vi "init stack.vi"() -> ()   [LabVIEW 2018]
uses:
  <vilib>/myRIO/Instrument Drivers/Onboard IO/AI/typedefs/AI Reference.ctl
  <vilib>/myRIO/Common/Instrument Driver Framework/Utilities/typedefs/myRIO Generic Hardware Reference.ctl
  <vilib>/myRIO/Common/Instrument Driver Framework/Utilities/typedefs/Hardware Version Enum.ctl
  <vilib>/myRIO/Common/Instrument Driver Framework/Utilities/typedefs/myRIO v1.0 Reference.ctl
  <vilib>/myRIO/Common/Instrument Driver Framework/Utilities/typedefs/Generic FPGA Reference.ctl
  <vilib>/myRIO/Common/Instrument Driver Framework/myRIO v1.0/AI/typedefs/AI Channels List.ctl
  <vilib>/myRIO/Common/Instrument Driver Framework/myRIO v1.0/AI/typedefs/AI Channels Enum.ctl
  <vilib>/myRIO/Common/Instrument Driver Framework/Utilities/typedefs/Analog Scaling Constants List.ctl
  <vilib>/myRIO/Common/Instrument Driver Framework/Utilities/typedefs/Analog Scaling Constants.ctl
  <vilib>/userdefined/High Color/nirio_resource_hc.ctl
  <vilib>/myRIO/Common/Instrument Driver Framework/Utilities/vis/Is FPGA Ref Available.vi
  <vilib>/myRIO/Common/Instrument Driver Framework/myRIO v1.0/AI/vis/myRIO v1.1 Open AI.vi
  <vilib>/myRIO/Instrument Drivers/Onboard IO/AI/vis/Read.vi
  <vilib>/myRIO/Common/Instrument Driver Framework/Utilities/vis/Validate Channels.vi
  <vilib>/myRIO/Common/Instrument Driver Framework/myRIO v1.0/AI/vis/myRIO v1.0 Reserve AI.vi
  <vilib>/myRIO/Common/Instrument Driver Framework/myRIO v1.0/AI/vis/myRIO v1.0 Build MUX Configuration AI.vi
  <vilib>/myRIO/Common/Instrument Driver Framework/myRIO v1.0/Resource Manager/vis/myRIO v1.0 Reserve Channel List.vi
  <vilib>/myRIO/Common/Instrument Driver Framework/myRIO v1.0/Resource Manager/vis/myRIO v1.0 Reserve Channel.vi
  <vilib>/myRIO/Common/Instrument Driver Framework/myRIO v1.0/Resource Manager/vis/myRIO v1.0 Unreserve Channel.vi
  <vilib>/myRIO/Common/Instrument Driver Framework/myRIO v1.0/Resource Manager/vis/myRIO v1.0 Build Mutex Name.vi
  <vilib>/Utility/VariantDataType/GetNumericInfo.vi
  <vilib>/Utility/error.llb/Error Cluster From Error Code.vi
  <vilib>/myRIO/Common/Instrument Driver Framework/myRIO v1.0/myRIO v1.1 Open.vi
  <vilib>/myRIO/Common/Instrument Driver Framework/myRIO v1.0/AI/vis/myRIO v1.0 Get Scaling Constants AI.vi
  <vilib>/myRIO/Common/Instrument Driver Framework/Utilities/vis/IO Manager.vi
  <vilib>/myRIO/Common/Instrument Driver Framework/Utilities/vis/Configuration Manager.vi
  <vilib>/myRIO/Common/Instrument Driver Framework/myRIO v1.0/myRIO v1.0 Close.vi
  <vilib>/myRIO/Common/Instrument Driver Framework/myRIO v1.0/AI/vis/myRIO v1.0 Read AI.vi
  <vilib>/myRIO/Express VI/Onboard IO/AI/AI Express VI.xnode
  <vilib>/myRIO/Instrument Drivers/Onboard IO/AI/vis/myRIO AI Open.xnode
  <vilib>/myRIO/Instrument Drivers/Onboard IO/AI/AI.lvlib
panel:
  out "Encoder Output 4":i32
  out "Encoder Output 3":i32
  out "Encoder Output 2":i32
  out "Encoder Output":i32
  in  "stop":bool
  out "diff":dbl
  out "right read":dbl
  out "left read":dbl
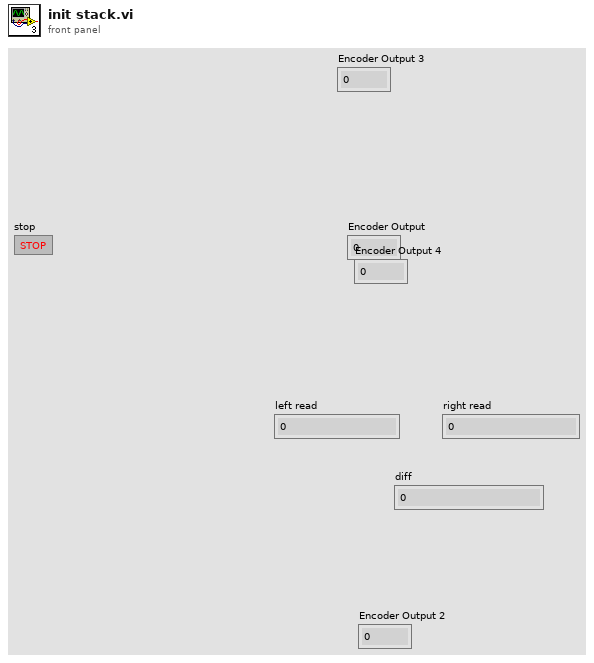
[diagram p1: front panel]
types:
  T1 = typedef "AI.lvlib/AI Reference.ctl" = cluster{"myRIO Reference":T2, "AI Channels List":T6, "AI Scaling Constants List":T8}
  T2 = typedef "myRIO Generic Hardware Reference.ctl" = cluster{"myRIO Model":T3, "myRIO Hardware Reference":T4}
  T3 = typedef "Hardware Version Enum.ctl" = enum16{"Unknown", "myRIO-1900", "myRIO-1950", "roboRIO", "NI ELVIS RIO CM", "ELVIS III"}
  T4 = typedef "myRIO v1.0 Reference.ctl" = cluster{"Generic FPGA Reference":T5, "Allow multiple opens":bool}
  T5 = typedef "Generic FPGA Reference.ctl" = refnum<k20>
  T6 = typedef "AI Channels List.ctl" = T7[]
  T7 = typedef "AI Channels Enum.ctl" = enum16{"Not Connected", "AudioIn/Left", "AudioIn/Right", "C/AI0", "C/AI1", "A/AI0", "A/AI1", "A/AI2", "A/AI3", "A/AI4", "A/AI5", "A/AI6", "A/AI7", "B/AI0", "B/AI1", "B/AI2", "B/AI3", "B/AI4", "B/AI5", "B/AI6", "B/AI7", "AI/AI0", "AI/AI1", "AI/AI2", "AI/AI3", "A/AI0 (DIFF)", "A/AI1 (DIFF)", "A/AI2 (DIFF)", "A/AI3 (DIFF)", "B/AI0 (DIFF)", "B/AI1 (DIFF)", "B/AI2 (DIFF)", "B/AI3 (DIFF)"}
  T8 = typedef "Analog Scaling Constants List.ctl" = T9[]
  T9 = typedef "Analog Scaling Constants.ctl" = cluster{"LSB Weight (Volts)":dbl, "Offset (Volts)":dbl, "Signed?":bool}
  T10 = typedef "nirio_resource_hc.ctl" = tag
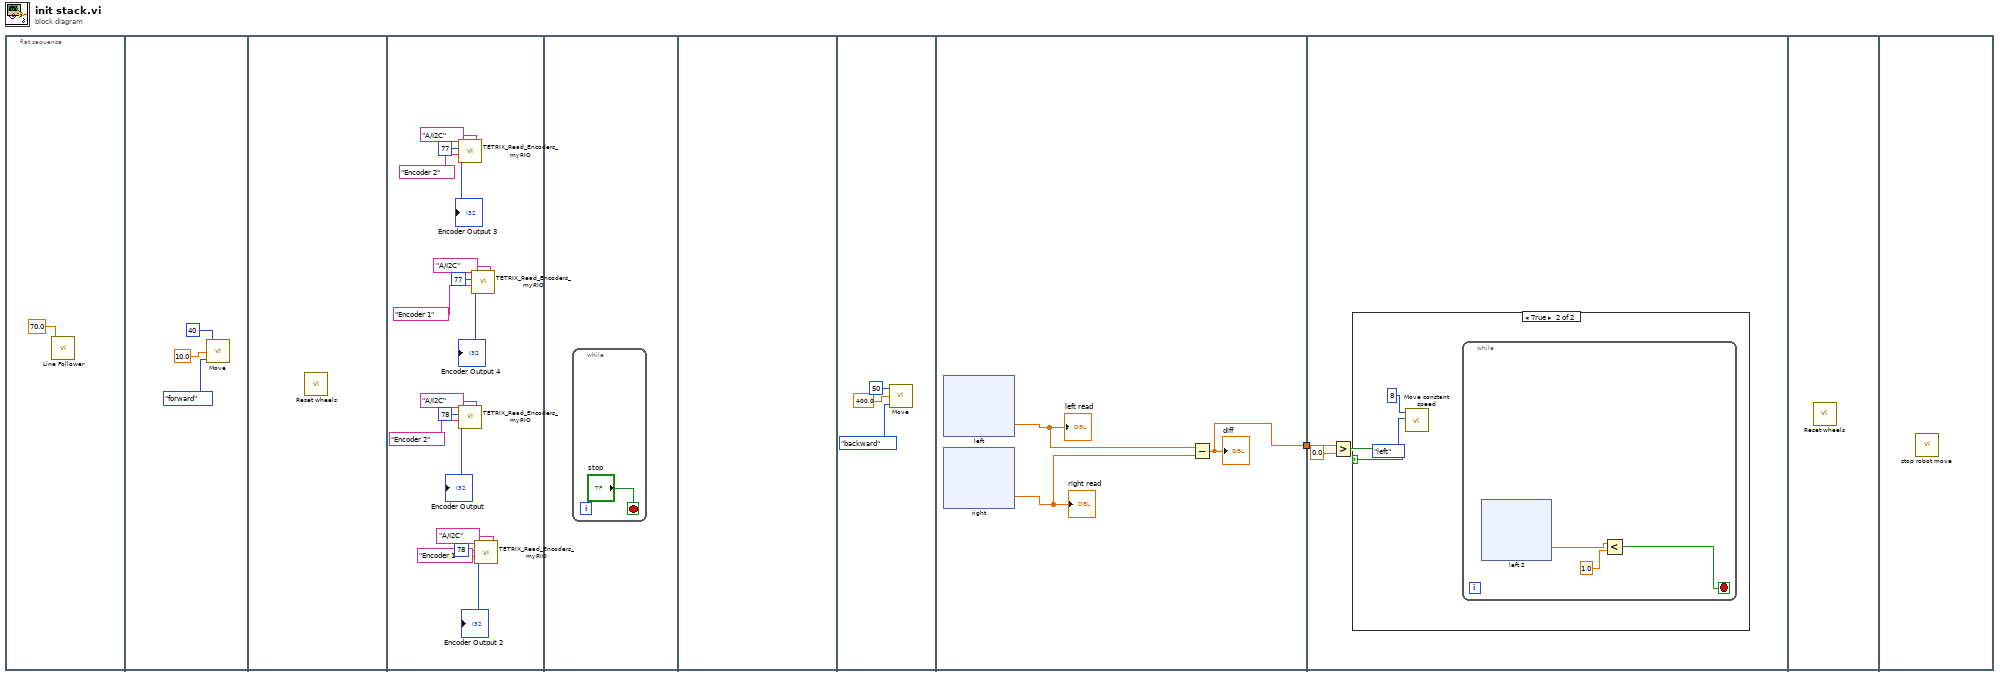
[diagram p0: block diagram]
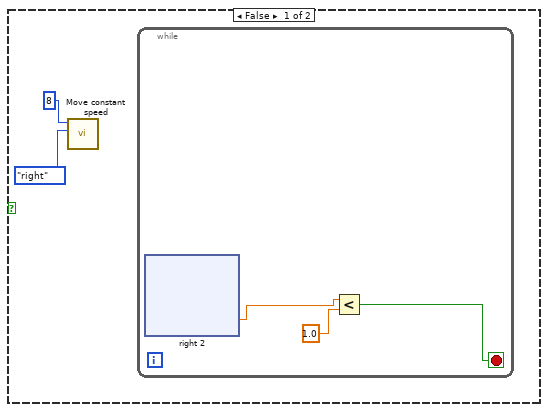
[diagram p2: hidden frame]
diagram:
  n1 = flat-sequence {
    tunnel: [w26] -> w1
    tunnel: w1 -> [w105]
    frame #0 {
      n2 = call "Line Follower.vi"("speed"=70.0) -> ()  [unwired: 11 in]
    }
    frame #1 {
      n3 = call "Move.vi"("Enum"=enum16{"forward", "backward", "left", "right"}."forward", "distance"=10.0, "speed"=40) -> ()  [unwired: 1 in]
    }
    frame #2 {
      n4 = call "Reset wheels.vi"() -> ()  [unwired: 12 in]
    }
    frame #3 {
      n5 = call <vilib>:"TETRIX_Read_Encoders_myRIO.vi"("myRIO MXP Port A/B"=tag "A/I2C", "Select Encoder"="Encoder 2", "Controller ID#  (I2C Address)"=u8 77) -> ("Encoder Output"=→"Encoder Output 3":i32)  [unwired: 3 in, 1 out]
      n6 = call <vilib>:"TETRIX_Read_Encoders_myRIO.vi"("myRIO MXP Port A/B"=tag "A/I2C", "Select Encoder"="Encoder 2", "Controller ID#  (I2C Address)"=u8 78) -> ("Encoder Output"=→"Encoder Output":i32)  [unwired: 3 in, 1 out]
      n7 = call <vilib>:"TETRIX_Read_Encoders_myRIO.vi"("myRIO MXP Port A/B"=tag "A/I2C", "Select Encoder"="Encoder 1", "Controller ID#  (I2C Address)"=u8 77) -> ("Encoder Output"=→"Encoder Output 4":i32)  [unwired: 3 in, 1 out]
      n8 = call <vilib>:"TETRIX_Read_Encoders_myRIO.vi"("myRIO MXP Port A/B"=tag "A/I2C", "Select Encoder"="Encoder 1", "Controller ID#  (I2C Address)"=u8 78) -> ("Encoder Output"=→"Encoder Output 2":i32)  [unwired: 3 in, 1 out]
    }
    frame #4 {
      n9 = while {
        stop <- "stop" stop-if-true
      }
    }
    frame #5 {
    }
    frame #6 {
      n10 = call "Move.vi"("Enum"=enum16{"forward", "backward", "left", "right"}."backward", "distance"=400.0, "speed"=50) -> ()  [unwired: 1 in]
    }
    frame #7 {
      n11 = xnode "left"() -> ("A/AI0 (Pin 3)"=w28:dbl)  [unwired: 1 in, 1 out]
      "left read" <- w28
      n12 = xnode "right"() -> ("A/AI1 (Pin 5)"=w27:dbl)  [unwired: 1 in, 1 out]
      "right read" <- w27
      n13 = Subtract(x=w28, y=w27) -> (x-y=w26:dbl)
      "diff" <- w26
    }
    frame #8 {
      n14 = Greater?(x=w105, y=0.0) -> (0:w103:bool)
      n15 = case shown="True" w103 {
        frame False {
          n16 = call "Move constant speed.vi"("Enum"=enum16{"forward", "backward", "left", "right"}."right", "speed"=8) -> ()  [unwired: 10 in]
          n17 = while {
            stop <- w109 stop-if-true
            n18 = xnode "right 2"() -> ("A/AI1 (Pin 5)"=w108:dbl)  [unwired: 1 in, 1 out]
            n19 = Less?(x=w108, y=1.0) -> (x < y?=w109:bool)
          }
        }
        frame True {
          n20 = call "Move constant speed.vi"("Enum"=enum16{"forward", "backward", "left", "right"}."left", "speed"=8) -> ()  [unwired: 10 in]
          n21 = while {
            stop <- w150 stop-if-true
            n22 = xnode "left 2"() -> ("A/AI0 (Pin 3)"=w152:dbl)  [unwired: 1 in, 1 out]
            n23 = Less?(x=w152, y=1.0) -> (x < y?=w150:bool)
          }
        }
      }
    }
    frame #9 {
      n24 = call "Reset wheels.vi"() -> ()  [unwired: 12 in]
    }
    frame #10 {
      n25 = call "stop robot move.vi"() -> ()  [unwired: 12 in]
    }
  }
